vi "Voltage - Continuous Input.vi"() -> ()   [LabVIEW 2014]
doc: "该范例演示了如果使用DAQmx设备连续采集带缓冲的电压信号。\n\n关于如何连接信号至DAQ设备，请查看设备文档。"
uses:
  <vilib>/DAQmx/create/channels.llb/DAQmx Create Channel (AI-Voltage-Basic).vi
  <vilib>/DAQmx/configure/timing.llb/DAQmx Timing (Sample Clock).vi
  <vilib>/DAQmx/configure/task.llb/DAQmx Configure Logging (TDMS).vi
  <vilib>/DAQmx/read.llb/DAQmx Read (Analog 1D Wfm NChan NSamp).vi
  <resource>/objmgr/daqmx.rc
panel:
  in  "停止":bool
  out "波形图":waveform(dbl)[](graph)
  in  "TDMS文件路径":path
  in  "每个循环采样点":i32=1000
  in  "采样率":dbl=1000.0
  in  "采样时钟源":tag="OnboardClock"
  in  "接线端配置":i32(ring)=-1 items=["默认值"=-1, "RSE"=10083, "NRSE"=10078, "差分"=10106, "伪差分"=12529]
  in  "最大电压":dbl=5.0
  in  "最小电压":dbl=-5.0
  in  "物理通道":tag="Dev1/ai0"
  out "实际采样率":dbl=1000.0 format="%0.2f"
  in  "记录模式":i32(ring)=10231 items=["关"=10231, "记录并读取"=15842]
  # "通道设置"
  # "采集数据"
  # "定时设置"
  # "记录设置"
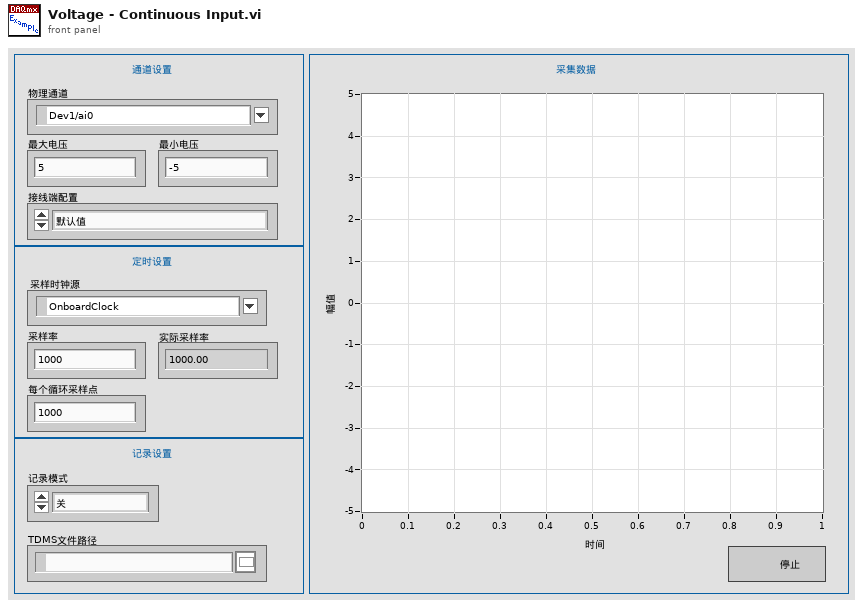
[diagram p1: front panel]
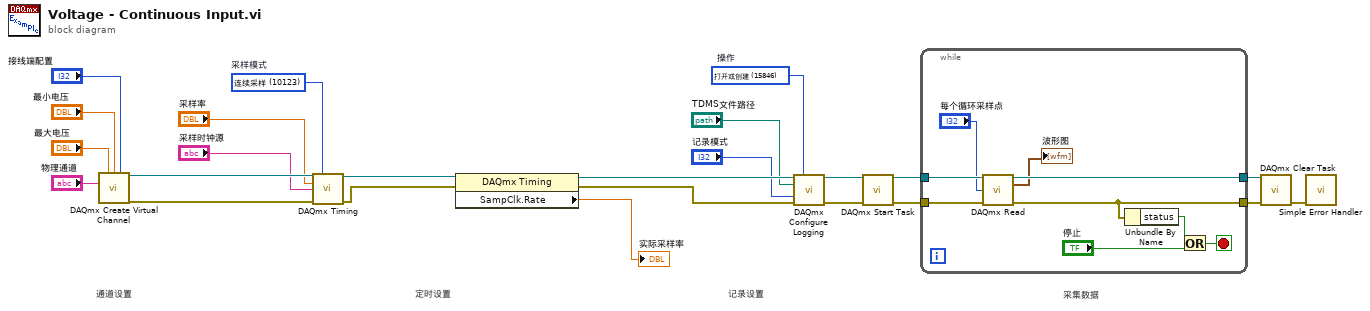
[diagram p0: block diagram]
diagram:
  w17 = 15846 items=["打开"=10437, "打开或创建"=15846, "创建或替换"=15847, "创建"=15848]  # 操作
  w22 = 10123 items=["有限采样"=10178, "连续采样"=10123, "硬件定时单点"=12522]  # 采样模式
  # "采集数据"
  # "定时设置"
  # "通道设置"
  # "记录设置"
  n1 = call-poly <vilib>:"DAQmx Create Virtual Channel.vi"("maximum value"="最大电压", "minimum value"="最小电压", "input terminal configuration"="接线端配置", "physical channels"="物理通道") -> ("task out"=w20:refnum<k21>, "error out"=w21:errorcluster)  [unwired: 10 in]
  n2 = call-poly <vilib>:"DAQmx Timing.vi"("task/channels in"=w20, "sample mode"=w22, "rate"="采样率", "source"="采样时钟源", "error in"=w21) -> ("task out"=w24:refnum<k21>, "error out"=w23:errorcluster)  [unwired: 9 in]
  n3 = property class="DAQmx Timing"(reference=w24, error in=w23) -> (reference out=w19:refnum<k21>, error out=w18:errorcluster, "SampClk.Rate"=→"实际采样率":dbl)
  n4 = call-poly <vilib>:"DAQmx Configure Logging.vi"("task/channels in"=w19, "operation"=w17, "file path"="TDMS文件路径", "logging mode"="记录模式", "error in"=w18) -> ("task out"=w2:refnum<k21>, "error out"=w1:errorcluster)  [unwired: 9 in]
  n5 = call <vilib>:"DAQmx Start Task.vi"("task/channels in"=w2, "error in"=w1) -> ("task out"=w16:refnum<k21>, "error out"=w15:errorcluster)  [unwired: 12 in]
  n6 = while {
    tunnel: w16 -> [w33]
    tunnel: w15 -> [w32]
    tunnel: [w29] -> w13
    tunnel: [w30] -> w14
    stop <- w31 stop-if-true
    n7 = call-poly <vilib>:"DAQmx Read.vi"("task/channels in"=w33, "number of samples per channel"="每个循环采样点", "error in"=w32) -> ("task out"=w30:refnum<k21>, "data"=→"波形图":waveform(dbl)[], "error out"=w29:errorcluster)  [unwired: 10 in]
    n8 = Unbundle By Name(w29) -> ("status"=w28:bool)
    n9 = Or(x=w28, y="停止") -> (x .or. y?=w31:bool)
  }
  n10 = call <vilib>:"DAQmx Clear Task.vi"("task in"=w14, "error in"=w13) -> ("error out"=w12:errorcluster)  [unwired: 13 in]
  n11 = call <vilib>:"Simple Error Handler.vi"("error in (no error)"=w12) -> ()  [unwired: 4 in, 5 out]
